vi "01 - Exemple - SyncSum.vi"() -> ()   [LabVIEW 2016]
uses:
  Library/DemoSkeleton/DemoSkeleton.lvlib
panel:
  out "Sum":i32
  in  "B":i32=2
  in  "A":i32=1
  # "+"
  # "="
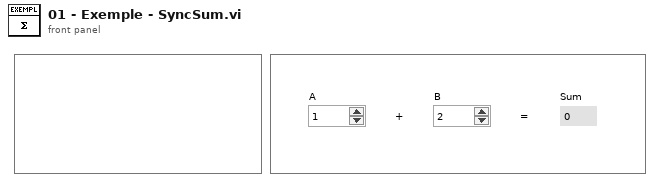
[diagram p1: front panel]
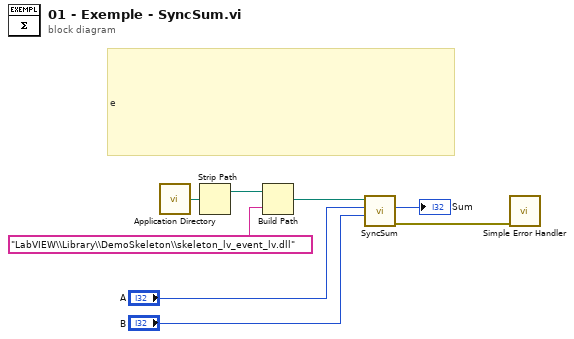
[diagram p0: block diagram]
diagram:
  # "e"
  n1 = call <vilib>:"Application Directory.vi"() -> ("Application Directory"=w4:path)
  n2 = Strip Path(path=w4) -> (stripped path=w3:path)  [unwired: 1 out]
  n3 = Build Path(base path=w3, name or relative path="LabVIEW\\Library\\DemoSkeleton\\skeleton_lv_event_lv.dll") -> (appended path=w1:path)
  n4 = call "SyncSum.vi"("B"="B", "A"="A", "path in"=w1) -> ("error out"=w8:errorcluster, "Sum"=→"Sum":i32)  [unwired: 6 in, 1 out]
  n5 = call <vilib>:"Simple Error Handler.vi"("error in (no error)"=w8) -> ()  [unwired: 4 in, 5 out]
